vi "initalise.vi"(8 "error in (no error)":errorcluster) -> (0 "error out":errorcluster, 3 "FileSystem out":refnum<class "FileSystem.lvclass">)   [LabVIEW 2011, in "Tools.lvlib" / "Filing.lvlib" / "FileSystem.lvclass"]
uses:
  FileSystem.lvclass
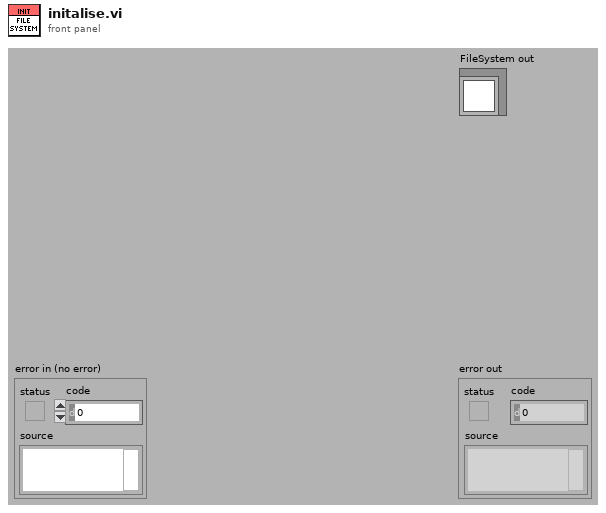
[diagram p1: front panel]
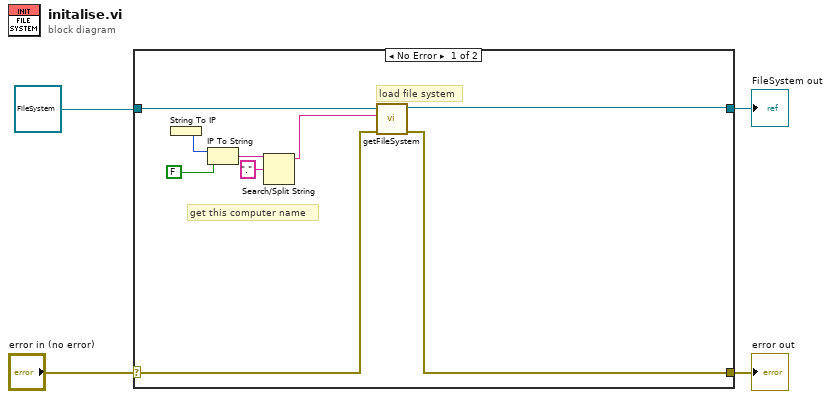
[diagram p0: block diagram]
diagram:
  n1 = case shown="No Error" "error in (no error)" {
    selector: "error in (no error)" -> [w12 w15]
    tunnel: [w11 w15] -> w3
    tunnel: [w10 w14] -> w2
    tunnel: refnum<class "FileSystem.lvclass"> refnum ("Tools.lvlib:Filing.lvlib:FileSystem.lvclass") -> [w13 w14]
    frame No Error {
      # "load file system"
      # "get this computer name"
      n2 = String To IP() -> (0:w8:u32)  [unwired: 1 in]
      n3 = IP To String(1:FALSE, 2:w8) -> (0:w7:string)
      n4 = Search/Split String(string=w7, search string/char (-)=".") -> (substring before match=w5:string)  [unwired: 1 in, 2 out]
      n5 = call "getFileSystem.vi"("error in (no error)"=w12, "computer"=w5, "FileSystem in"=w13) -> ("error out"=w11:errorcluster, "FileSystem out"=w10:refnum<class "FileSystem.lvclass">)  [unwired: 7 in]
    }
    frame Error {
    }
  }
  "error out" <- w3
  "FileSystem out" <- w2
